vi "LPTSequenceBulilder.vi"(10 "Number Of Operations":i32, 11 "Proocessing Times MxJ":u16[][](array[numeric])) -> (2 "Falttened Processing Times":u16[](array[numeric]), 3 "LPT Sequence":i32[](array[numeric]))   [LabVIEW 2013]
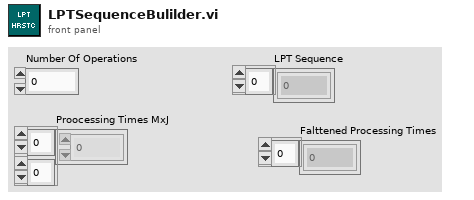
[diagram p1: front panel]
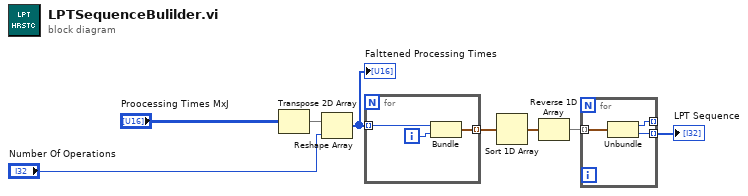
[diagram p0: block diagram]
diagram:
  n1 = Transpose 2D Array(2D array="Proocessing Times MxJ") -> (transposed array=w1:u16[][])
  n2 = Reshape Array(w1, "Number Of Operations") -> (w6:u16[])
  "Falttened Processing Times" <- w6
  n3 = for {
    tunnel: w6 -> [w11] mode=indexing
    tunnel: [w9] -> w3 mode=indexing
    i -> [w10]
    n4 = Bundle(w11, w10) -> (w9:cluster{u16, i32})  [unwired: 1 in]
  }
  n5 = Sort 1D Array(array=w3) -> (sorted array=w4:cluster{u16, i32}[])
  n6 = Reverse 1D Array(array=w4) -> (reversed array=w2:cluster{u16, i32}[])
  n7 = for {
    tunnel: w2 -> [w14] mode=indexing
    tunnel: [w13] -> _ mode=indexing
    tunnel: [w12] -> w7 mode=indexing
    n8 = Unbundle(w14) -> (w13:u16, w12:i32)
  }
  "LPT Sequence" <- w7
